vi "Draw Tree.vi"(8 "error in":errorcluster, 10 "Tree Control Items":T1(array[cluster]), 11 "TreeControl in":refnum<vi>) -> (0 "error out":errorcluster, 3 "TreeControl out":refnum<vi>)   [LabVIEW 2019, in "Panther Dashboard.lvlib"]
uses:
  Panther Dashboard.lvlib
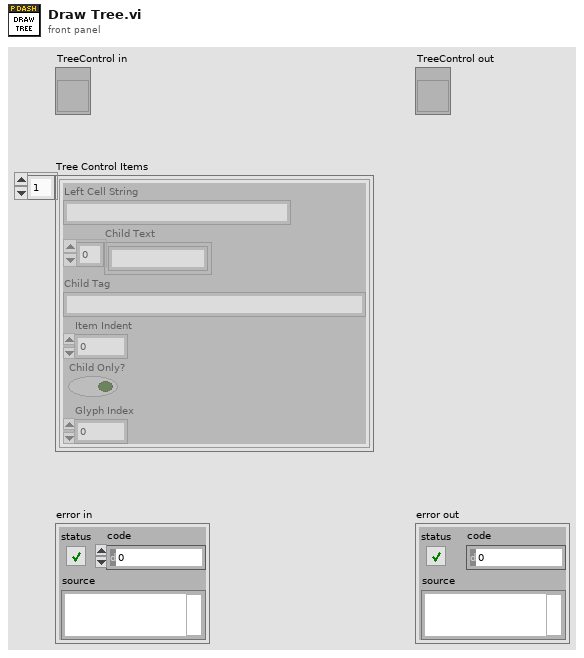
[diagram p1: front panel]
types:
  T1 = cluster{"Left Cell String":string, "Child Text":string[], "Child Tag":string, "Item Indent":i32, "Child Only?":bool, "Glyph Index":i32}[]
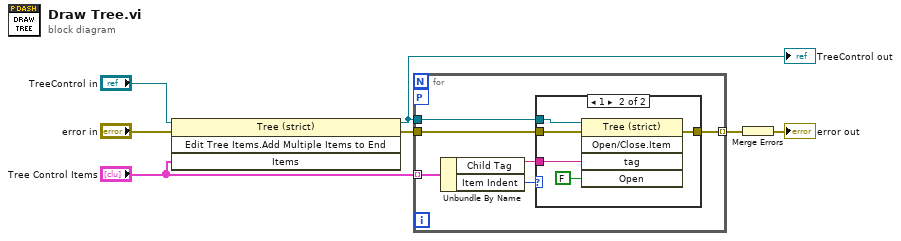
[diagram p0: block diagram]
diagram:
  n1 = invoke on="Invoke Node" class="Tree (strict)" method="Edit Tree Items.Add Multiple Items to End"(reference="TreeControl in", error in="error in", "Items"="Tree Control Items") -> (reference out=w1:refnum<vi>, error out=w6:errorcluster)  [unwired: 1 in, 2 out]
  "TreeControl out" <- w1
  n2 = for {
    tunnel: "Tree Control Items" -> [w10] mode=indexing
    tunnel: w1 -> [w11]
    tunnel: w6 -> [w13]
    tunnel: [w12] -> w4 mode=indexing
    workers-P: _ -> [_]
    n3 = Unbundle By Name(w10) -> ("Child Tag"=w8:string, "Item Indent"=w9:i32)
    n4 = case shown="1" w9 {
      tunnel: w13 -> [w14 w19]
      tunnel: [w14 w18] -> w12
      tunnel: w11 -> [_ w17]
      tunnel: w8 -> [_ w15]
      frame Default {
      }
      frame 1 {
        n5 = invoke class="Tree (strict)" method="Open/Close.Item"(reference=w17, error in=w19, "tag"=w15, "Open"=FALSE ("Open?")) -> (error out=w18:errorcluster)  [unwired: 1 in, 4 out]
      }
    }
  }
  n6 = Merge Errors(w4) -> (→"error out":errorcluster)
